vi "VSG25_AM.vi"(0 "Device Handle In":i32, 1 "Run as Subpanel":bool, 2 "AM Cluster In":T1={"Carrier Freq"=1.0, "Baseband Freq"=1.0, "Carrier Hz"=3, "Baseband Hz"=1, "Modulation Depth"=50.0, "Amplitude"=-10.0, "Modulation Shape"=0} {"Modulation Shape" items=["Sine Wave", "Triangle Wave", "Square Wave", "Ramp Wave"]; "Carrier Hz" items=["Hz", "kHz", "MHz", "GHz"]; "Baseband Hz" items=["Hz", "kHz", "MHz", "GHz"]}, 3 "Error In":errorcluster) -> (5 "Device Handle Out":i32, 6 "AM Cluster Out":T1 {"Modulation Shape" items=["Sine Wave", "Triangle Wave", "Square Wave", "Ramp Wave"]; "Carrier Hz" items=["Hz", "kHz", "MHz", "GHz"]; "Baseband Hz" items=["Hz", "kHz", "MHz", "GHz"]}, 7 "Error Out":errorcluster)   [LabVIEW 2014]
uses:
  Frequency Hertz.ctl
  Shape Control.ctl
  AM Cluster.ctl
  sg_lib/VSG25A.lvlib
panel:
  in  "Stop":bool
  out "Device Selected":bool
  in  "Modulation Shape":T3 items=["Sine Wave", "Triangle Wave", "Square Wave", "Ramp Wave"]
  in  "Modulation Depth":dbl
  in  "Baseband Hz":T2 items=["Hz", "kHz", "MHz", "GHz"]
  in  "Baseband Frequency":dbl
  in  "RF On":bool
  in  "Carrier Hz":T2 items=["Hz", "kHz", "MHz", "GHz"]
  in  "Amplitude (dBm)":dbl
  in  "Carrier Frequency":dbl
  # "Amplitude Modulation"
  # "( 1 to 99 %)"
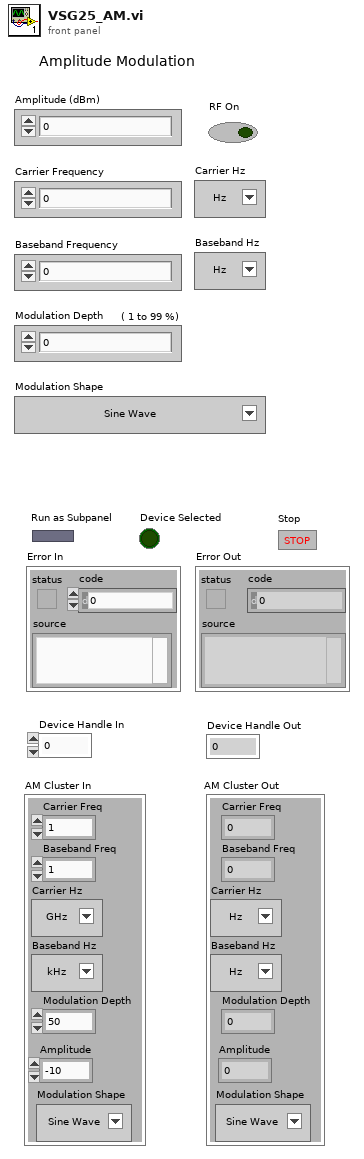
[diagram p1: front panel]
types:
  T1 = typedef "AM Cluster.ctl" = cluster{"Carrier Freq":dbl, "Baseband Freq":dbl, "Carrier Hz":T2, "Baseband Hz":T2, "Modulation Depth":dbl, "Amplitude":dbl, "Modulation Shape":T3}
  T2 = typedef "Frequency Hertz.ctl" = u16
  T3 = typedef "Shape Control.ctl" = u16
  T4 = enum16{"Init", "Proc Events", "Write VSG25", "Exit"}
  T5 = enum32{"Bad", "Idle", "Run top level", "Running"}
  T6 = enum16{"Check Amplitude ", "Check Carrier", "Check Baseband", "Check Modulation Depth", "Stop RF", "Set Freq and Amp", "Set AM", "Finish"}
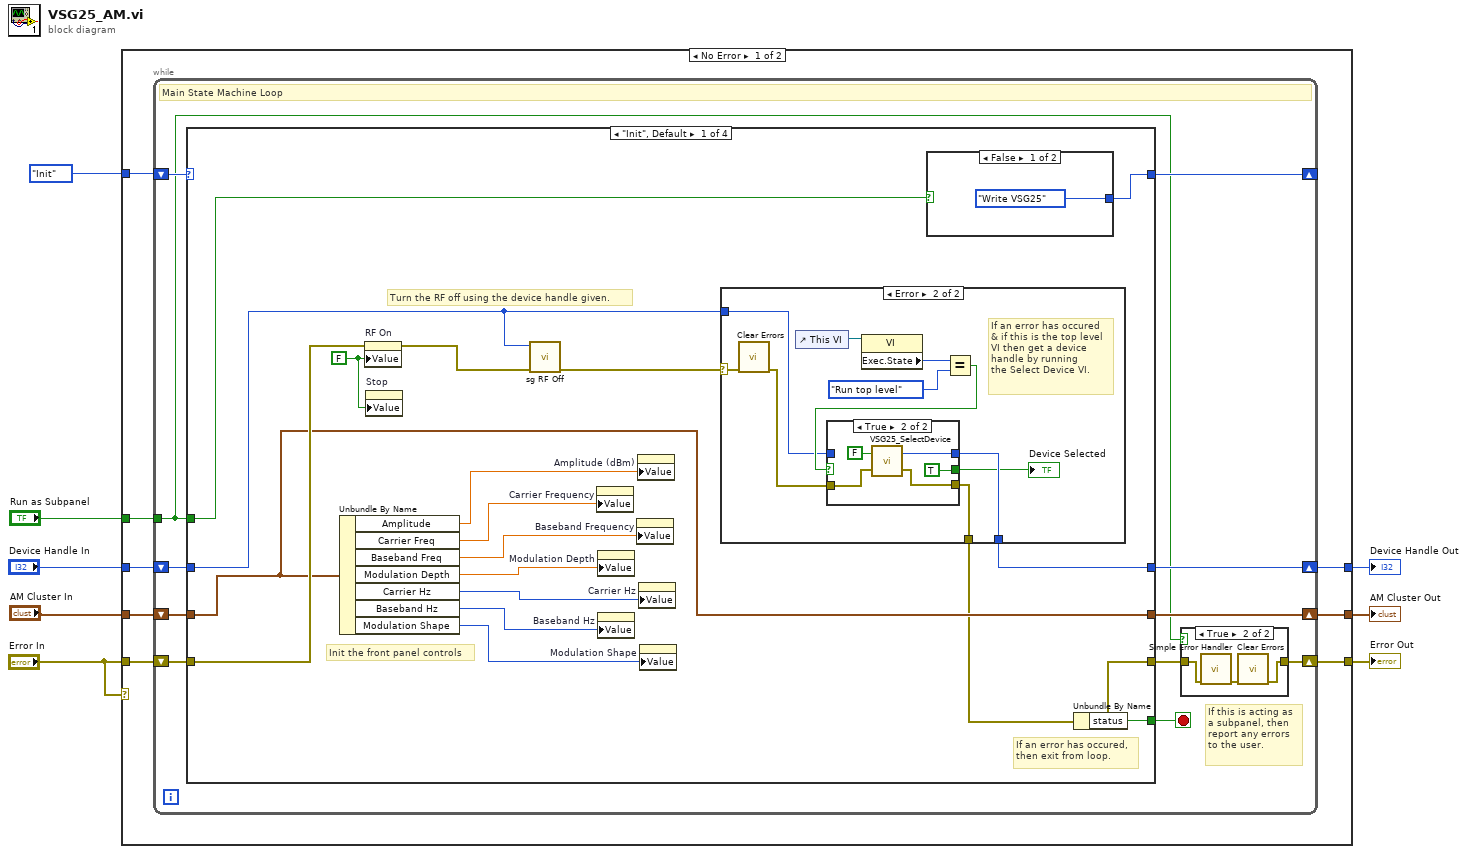
[diagram p0: block diagram]
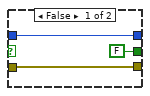
[diagram p4: hidden frame]
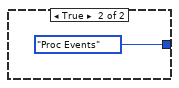
[diagram p5: hidden frame]
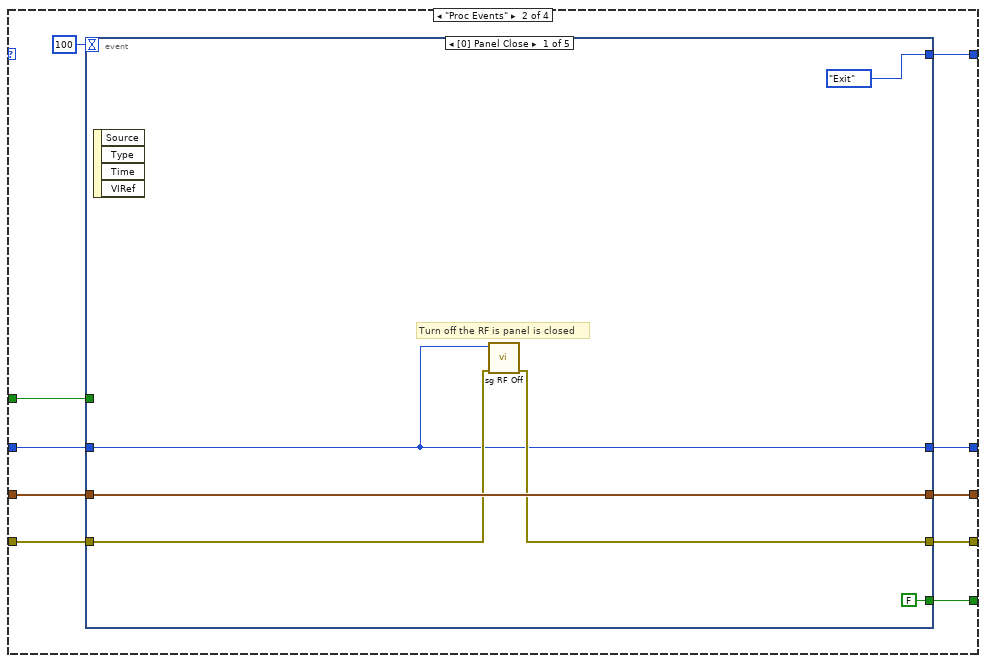
[diagram p6: hidden frame]
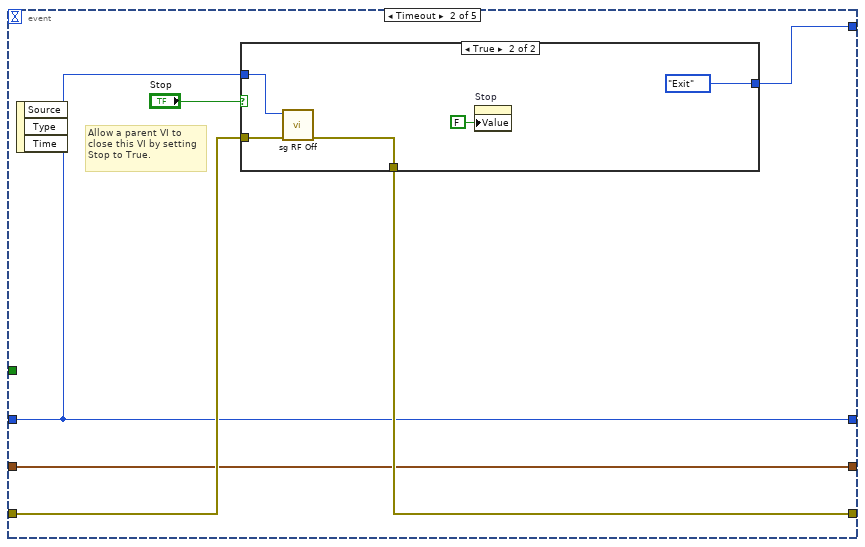
[diagram p7: hidden frame]
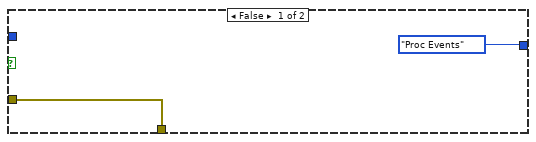
[diagram p8: hidden frame]
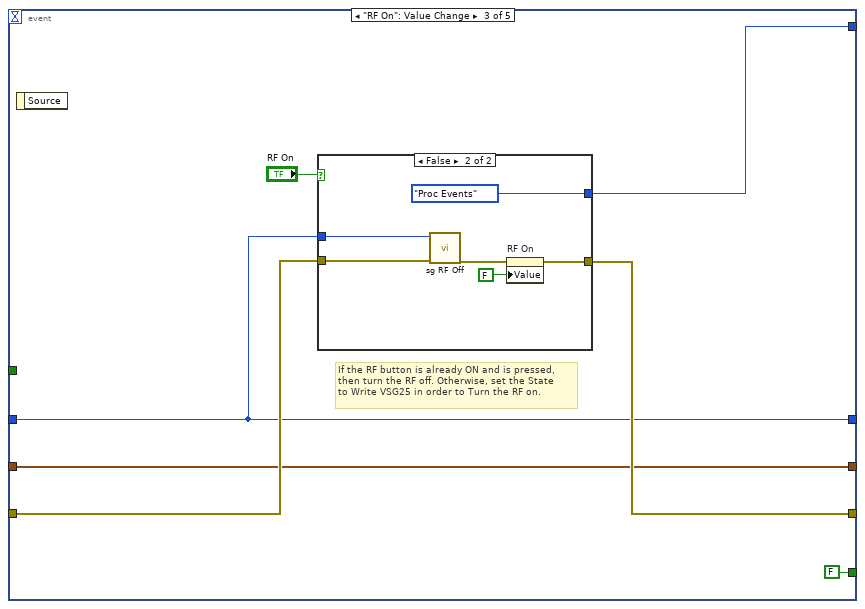
[diagram p9: hidden frame]
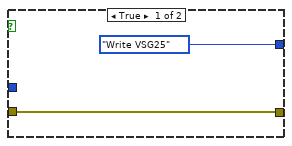
[diagram p10: hidden frame]
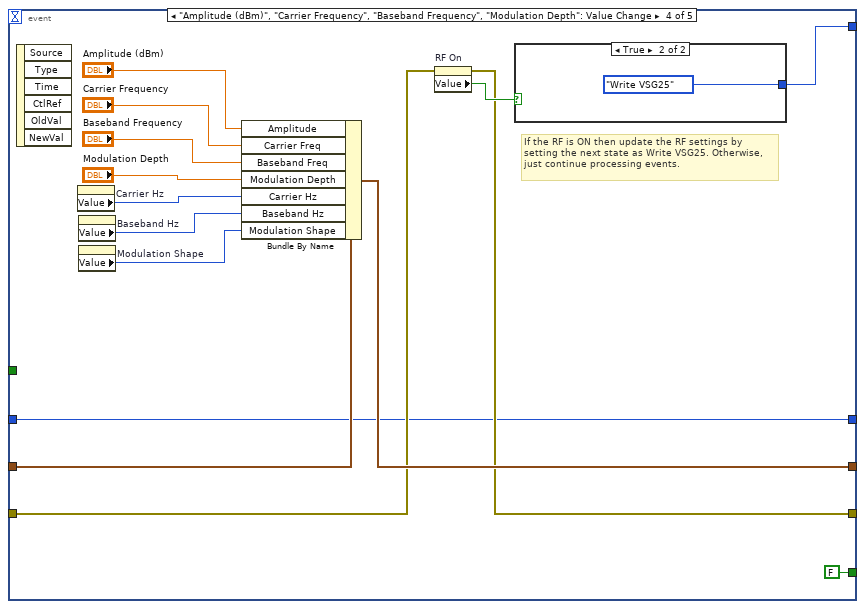
[diagram p11: hidden frame]
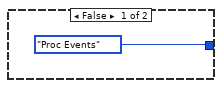
[diagram p12: hidden frame]
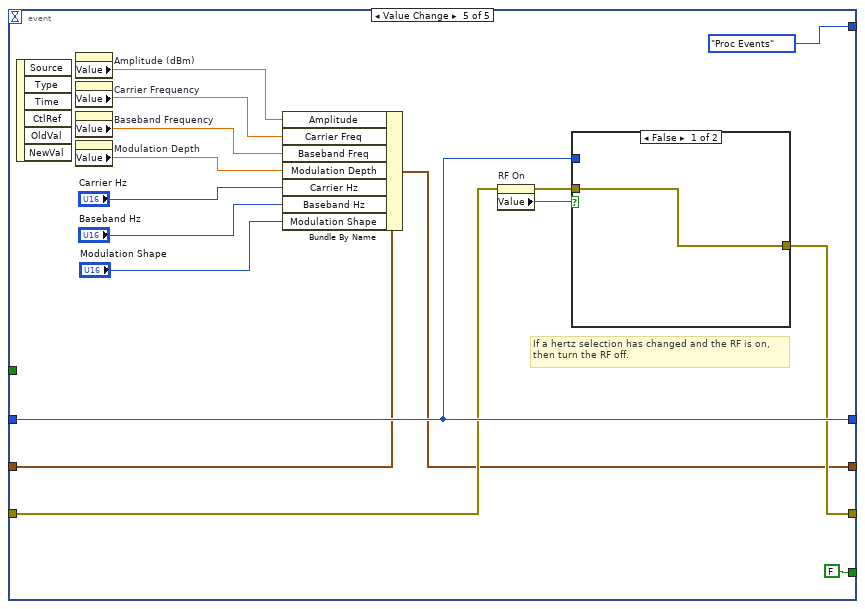
[diagram p13: hidden frame]
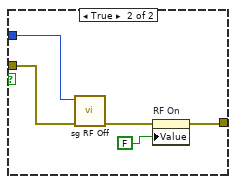
[diagram p14: hidden frame]
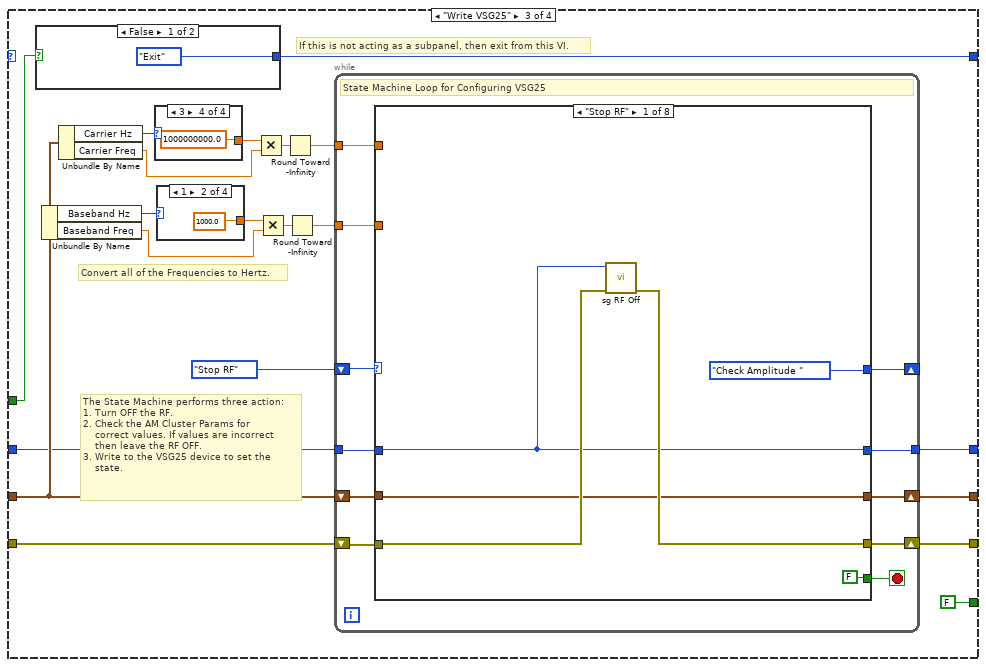
[diagram p15: hidden frame]
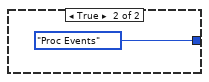
[diagram p16: hidden frame]
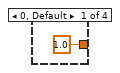
[diagram p17: hidden frame]
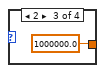
[diagram p18: hidden frame]
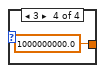
[diagram p19: hidden frame]
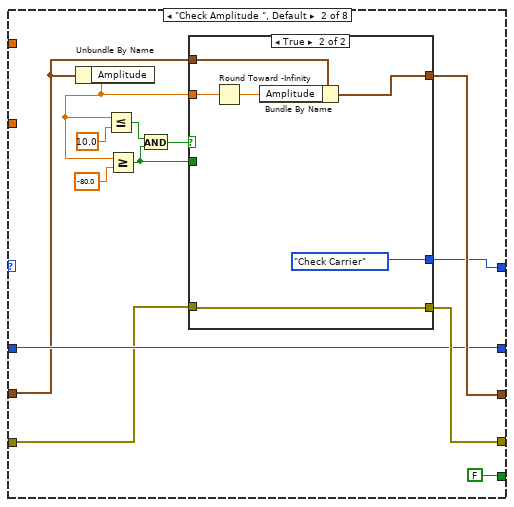
[diagram p20: hidden frame]
diagram:
  n1 = case shown="No Error" "Error In" {
    tunnel: "Error In" -> [w12 w323]
    tunnel: T4."Init" -> [w16 _]
    tunnel: "Run as Subpanel" -> [w15 _]
    tunnel: "Device Handle In" -> [w14 w321]
    tunnel: "AM Cluster In" -> [w13 w322]
    tunnel: [w11 w323] -> w4
    tunnel: [w10 w322] -> w1
    tunnel: [w9 w321] -> w3
    frame No Error {
      n2 = while {
        shift-right: [w26] -> _
        shift-left: w16 -> [w27]
        tunnel: w15 -> [w17]
        shift-right: [w18] -> w11
        shift-left: w12 -> [w23]
        shift-right: [w21] -> w10
        shift-left: w13 -> [w24]
        shift-right: [w20] -> w9
        shift-left: w14 -> [w25]
        stop <- w22 stop-if-true
        # "If this is acting as \na subpanel, then\nreport any errors\nto the user."
        # "Main State Machine Loop"
        n3 = case shown="\"Init\", Default" w27 {
          selector: w27 -> [_ _ _ w316]
          tunnel: [w42 w74 w157 w316] -> w26
          tunnel: w17 -> [w45 w78 w156 _]
          tunnel: w25 -> [w36 w79 w162 w311]
          tunnel: w24 -> [w43 w80 w163 w312]
          tunnel: w23 -> [w44 w81 w166 w313]
          tunnel: [w41 w75 FALSE TRUE] -> w22
          tunnel: [w37 w73 w161 w314] -> w19
          tunnel: [w43 w77 w160 w312] -> w21
          tunnel: [w38 w76 w159 w311] -> w20
          frame "Init", Default {
            w32 = FALSE ("RF On")
            # "Init the front panel controls"
            # "Turn the RF off using the device handle given."
            # "If an error has occured,\nthen exit from loop."
            n4 = Unbundle By Name(w43) -> ("Amplitude"=w49:dbl, "Carrier Freq"=w48:dbl, "Baseband Freq"=w47:dbl, "Modulation Depth"=w46:dbl, "Carrier Hz"=w35:T2, "Baseband Hz"=w34:T2, "Modulation Shape"=w33:T3)
            n5 = property on="RF On" class="Bool (strict)"(error in=w44, "Value"=w32) -> (error out=w40:errorcluster)  [unwired: 1 in, 1 out]
            n6 = property on="Stop" class="Bool (strict)"("Value"=w32) -> ()  [unwired: 2 in, 2 out]
            n7 = call "sg RF Off.vi"("error in (no error)"=w40, "device"=w36) -> ("error out"=w39:errorcluster)  [unwired: 8 in, 1 out]
            n8 = property on="Carrier Frequency" class="DigNum (strict)"("Value"=w48) -> ()  [unwired: 2 in, 2 out]
            n9 = property on="Modulation Depth" class="DigNum (strict)"("Value"=w46) -> ()  [unwired: 2 in, 2 out]
            n10 = property on="Baseband Hz" class="Ring (strict)"("Value"=w34) -> ()  [unwired: 2 in, 2 out]
            n11 = property on="Baseband Frequency" class="DigNum (strict)"("Value"=w47) -> ()  [unwired: 2 in, 2 out]
            n12 = property on="Amplitude (dBm)" class="DigNum (strict)"("Value"=w49) -> ()  [unwired: 2 in, 2 out]
            n13 = property on="Carrier Hz" class="Ring (strict)"("Value"=w35) -> ()  [unwired: 2 in, 2 out]
            n14 = property on="Modulation Shape" class="Ring (strict)"("Value"=w33) -> ()  [unwired: 2 in, 2 out]
            n15 = case shown="Error" w39 {
              selector: w39 -> [w50 w57]
              tunnel: [w51 w55] -> w38
              tunnel: [w50 w54] -> w37
              tunnel: w36 -> [w51 w53]
              frame No Error {
              }
              frame Error {
                # "If an error has occured\n& if this is the top level\nVI then get a device\nhandle by running \nthe Select Device VI."
                n16 = call <vilib>:"Clear Errors.vi"("error in (no error)"=w57) -> ("error out"=w56:errorcluster)  [unwired: 5 in, 1 out]
                n17 = control-ref of="This VI"() -> (w61:refnum<vi>)
                n18 = property class="VI"(reference=w61) -> ("Exec.State"=w60:T5)  [unwired: 1 in, 2 out]
                n19 = Equal?(x=w60, y=T5."Run top level" ("Execution:State 2")) -> (x = y?=w58:bool)
                n20 = case shown="True" w58 {
                  tunnel: [w64 w69] -> w55
                  tunnel: w53 -> [w64 _]
                  tunnel: w56 -> [w63 w67]
                  tunnel: [w63 w66] -> w54
                  tunnel: [FALSE TRUE] -> w52
                  frame False {
                  }
                  frame True {
                    n21 = call "VSG25_SelectDevice.vi"("ErrorIn"=w67, "AutoSel"=FALSE) -> ("ErrorOut"=w66:errorcluster, "deviceHandle"=w69:i32)
                  }
                }
                "Device Selected" <- w52
              }
            }
            n22 = case shown="False" w45 {
              tunnel: [T4."Write VSG25" T4."Proc Events"] -> w42
              frame False {
              }
              frame True {
              }
            }
            n23 = Unbundle By Name(w37) -> ("status"=w41:bool)
          }
          frame "Proc Events" {
            n24 = event shown="[0] Panel Close" {
              selector: _ -> [_ _ _ _ _]
              dyn-events: _ -> [_ _ _ _ _]
              timeout: 100 -> [_ _ _ _ _]
              tunnel: w81 -> [w84 w93 w106 w120 w144]
              tunnel: w80 -> [w85 w91 w104 w130 w143]
              tunnel: w79 -> [w82 w90 w103 w118 w146]
              tunnel: w78 -> [_ _ _ _ _]
              tunnel: [w83 w92 w105 w119 w145] -> w73
              tunnel: [w85 w91 w104 w129 w142] -> w77
              tunnel: [w82 w90 w103 w118 w146] -> w76
              tunnel: [FALSE _ FALSE FALSE FALSE] -> w75
              tunnel: [T4."Exit" w88 w102 w121 T4."Proc Events"] -> w74
              event Panel Close {
                # "Turn off the RF is panel is closed"
                n25 = event-data() -> ()  [unwired: 1 in, 4 out]
                n26 = call "sg RF Off.vi"("error in (no error)"=w84, "device"=w82) -> ("error out"=w83:errorcluster)  [unwired: 8 in, 1 out]
              }
              event Timeout {
                # "Allow a parent VI to \nclose this VI by setting\nStop to True."
                n27 = event-data() -> ()  [unwired: 1 in, 3 out]
                n28 = case shown="True" "Stop" {
                  tunnel: w93 -> [w95 w100]
                  tunnel: [w95 w99] -> w92
                  tunnel: w90 -> [_ w98]
                  tunnel: [T4."Proc Events" T4."Exit"] -> w88
                  frame False {
                  }
                  frame True {
                    n29 = call "sg RF Off.vi"("error in (no error)"=w100, "device"=w98) -> ("error out"=w99:errorcluster)  [unwired: 8 in, 1 out]
                    n30 = property on="Stop" class="Bool (strict)"("Value"=FALSE ("Stop")) -> ()  [unwired: 2 in, 2 out]
                  }
                }
              }
              event "RF On": Value Change {
                # "If the RF button is already ON and is pressed, \nthen turn the RF off. Otherwise, set the State\nto Write VSG25 in order to Turn the RF on."
                n31 = event-data() -> ()  [unwired: 1 in, 1 out]
                n32 = case shown="False" "RF On" {
                  tunnel: [w108 w113] -> w105
                  tunnel: w106 -> [w108 w115]
                  tunnel: w103 -> [_ w114]
                  tunnel: [T4."Write VSG25" T4."Proc Events"] -> w102
                  frame True {
                  }
                  frame False {
                    n33 = call "sg RF Off.vi"("error in (no error)"=w115, "device"=w114) -> ("error out"=w112:errorcluster)  [unwired: 8 in, 1 out]
                    n34 = property on="RF On" class="Bool (strict)"(error in=w112, "Value"=FALSE ("RF On")) -> (error out=w113:errorcluster)  [unwired: 1 in, 1 out]
                  }
                }
              }
              event "Amplitude (dBm)", "Carrier Frequency", "Baseband Frequency", "Modulation Depth": Value Change {
                # "If the RF is ON then update the RF settings by\nsetting the next state as Write VSG25. Otherwise,\njust continue processing events."
                n35 = event-data() -> ()  [unwired: 1 in, 6 out]
                n36 = property on="Carrier Hz" class="Ring (strict)"() -> ("Value"=w124:T2)  [unwired: 2 in, 2 out]
                n37 = property on="Baseband Hz" class="Ring (strict)"() -> ("Value"=w123:T2)  [unwired: 2 in, 2 out]
                n38 = property on="Modulation Shape" class="Ring (strict)"() -> ("Value"=w116:T3)  [unwired: 2 in, 2 out]
                n39 = Bundle By Name(cluster=w130, "Amplitude"="Amplitude (dBm)", "Carrier Freq"="Carrier Frequency", "Baseband Freq"="Baseband Frequency", "Modulation Depth"="Modulation Depth", "Carrier Hz"=w124, "Baseband Hz"=w123, "Modulation Shape"=w116) -> (w129:T1)
                n40 = property on="RF On" class="Bool (strict)"(error in=w120) -> (error out=w119:errorcluster, "Value"=w122:bool)  [unwired: 1 in, 1 out]
                n41 = case shown="True" w122 {
                  tunnel: [T4."Proc Events" T4."Write VSG25"] -> w121
                  frame False {
                  }
                  frame True {
                  }
                }
              }
              event Value Change {
                # "If a hertz selection has changed and the RF is on,\nthen turn the RF off."
                n42 = event-data() -> ()  [unwired: 1 in, 6 out]
                n43 = property on="Amplitude (dBm)" class="DigNum (strict)"() -> ("Value"=w141:dbl)  [unwired: 2 in, 2 out]
                n44 = property on="Carrier Frequency" class="DigNum (strict)"() -> ("Value"=w140:dbl)  [unwired: 2 in, 2 out]
                n45 = property on="Baseband Frequency" class="DigNum (strict)"() -> ("Value"=w139:dbl)  [unwired: 2 in, 2 out]
                n46 = property on="Modulation Depth" class="DigNum (strict)"() -> ("Value"=w138:dbl)  [unwired: 2 in, 2 out]
                n47 = Bundle By Name(cluster=w143, "Amplitude"=w141, "Carrier Freq"=w140, "Baseband Freq"=w139, "Modulation Depth"=w138, "Carrier Hz"="Carrier Hz", "Baseband Hz"="Baseband Hz", "Modulation Shape"="Modulation Shape") -> (w142:T1)
                n48 = property on="RF On" class="Bool (strict)"(error in=w144) -> (error out=w148:errorcluster, "Value"=w147:bool)  [unwired: 1 in, 1 out]
                n49 = case shown="False" w147 {
                  tunnel: [w149 w150] -> w145
                  tunnel: w148 -> [w149 w154]
                  tunnel: w146 -> [_ w153]
                  frame False {
                  }
                  frame True {
                    n50 = call "sg RF Off.vi"("error in (no error)"=w154, "device"=w153) -> ("error out"=w151:errorcluster)  [unwired: 8 in, 1 out]
                    n51 = property on="RF On" class="Bool (strict)"(error in=w151, "Value"=FALSE ("RF On")) -> (error out=w150:errorcluster)  [unwired: 1 in, 1 out]
                  }
                }
              }
            }
          }
          frame "Write VSG25" {
            # "If this is not acting as a subpanel, then exit from this VI."
            # "Convert all of the Frequencies to Hertz."
            # "The State Machine performs three action:\n1. Turn OFF the RF.\n2. Check the AM Cluster Params for \n    correct values. If values are incorrect\n    then leave the RF OFF.\n3. Write to the VSG25 device to set the\n    state."
            n52 = case shown="False" w156 {
              tunnel: [T4."Exit" T4."Proc Events"] -> w157
              frame False {
              }
              frame True {
              }
            }
            n53 = Unbundle By Name(w163) -> ("Baseband Hz"=w168:T2, "Baseband Freq"=w170:dbl)
            n54 = Unbundle By Name(w163) -> ("Carrier Hz"=w173:T2, "Carrier Freq"=w171:dbl)
            n55 = case shown="3" w173 {
              tunnel: [1.0 ("y") 1000.0 ("y") 1000000.0 ("y") 1000000000.0 ("y")] -> w172
              frame 0, Default {
              }
              frame 1 {
              }
              frame 2 {
              }
              frame 3 {
              }
            }
            n56 = case shown="1" w168 {
              tunnel: [1.0 ("y") 1000.0 ("y") 1000000.0 ("y") 1000000000.0 ("y")] -> w169
              frame 0, Default {
              }
              frame 1 {
              }
              frame 2 {
              }
              frame 3 {
              }
            }
            n57 = Multiply(x=w172, y=w171) -> (x*y=w174:dbl)
            n58 = Multiply(x=w169, y=w170) -> (x*y=w167:dbl)
            n59 = Round Toward -Infinity(1:w174) -> (0:w165:dbl)
            n60 = Round Toward -Infinity(1:w167) -> (0:w164:dbl)
            n61 = while {
              shift-right: [w183] -> _
              shift-left: T6."Stop RF" -> [w191]
              tunnel: w165 -> [w184]
              tunnel: w164 -> [w181]
              tunnel: w162 -> [w185]
              tunnel: [w182] -> w159
              shift-right: [w187] -> w161
              shift-left: w166 -> [w189]
              shift-right: [w186] -> w160
              shift-left: w163 -> [w190]
              stop <- w188 stop-if-true
              # "State Machine Loop for Configuring VSG25"
              n62 = case shown="\"Stop RF\"" w191 {
                selector: w191 -> [_ _ _ _ _ _ _ w299]
                tunnel: w190 -> [w194 w200 w228 w248 w265 w284 w291 w301]
                tunnel: w189 -> [w196 w199 w231 w250 w269 w286 w297 w302]
                tunnel: [FALSE FALSE FALSE FALSE FALSE FALSE FALSE TRUE] -> w188
                tunnel: [w195 w203 w230 w247 w267 w283 w296 w302] -> w187
                tunnel: [w194 w202 w228 w248 w265 w284 w291 w301] -> w186
                tunnel: w185 -> [w193 w201 w227 w249 w268 w285 w293 w300]
                tunnel: [w193 w201 w227 w249 w268 w285 w293 w300] -> w182
                tunnel: w184 -> [_ _ w233 _ _ w287 _ _]
                tunnel: [T6."Check Amplitude " w198 w232 w246 w266 T6."Set AM" T6."Finish" w299] -> w183
                tunnel: w181 -> [_ _ _ w251 _ _ w294 _]
                frame "Stop RF" {
                  n63 = call "sg RF Off.vi"("error in (no error)"=w196, "device"=w193) -> ("error out"=w195:errorcluster)  [unwired: 8 in, 1 out]
                }
                frame "Check Amplitude ", Default {
                  n64 = Unbundle By Name(w200) -> ("Amplitude"=w205:dbl)
                  n65 = Less Or Equal?(x=w205, y=10.0) -> (x <= y?=w209:bool)
                  n66 = Greater Or Equal?(x=w205, y=-80.0) -> (x >= y?=w206:bool)
                  n67 = And(x=w209, y=w206) -> (x .and. y?=w210:bool)
                  n68 = case shown="True" w210 {
                    tunnel: w206 -> [w220 _]
                    tunnel: w205 -> [_ w225]
                    tunnel: w200 -> [w217 w224]
                    tunnel: [w216 w223] -> w202
                    tunnel: [T6."Finish" T6."Check Carrier"] -> w198
                    tunnel: w199 -> [w214 w222]
                    tunnel: [w212 w222] -> w203
                    frame False {
                      n69 = Select(t=10.0, s=w220, f=-80.0) -> (s? t:f=w215:dbl)
                      n70 = Bundle By Name(cluster=w217, "Carrier Freq"=w215) -> (w216:T1)
                      n71 = property on="Amplitude (dBm)" class="DigNum (strict)"("Value"=w215) -> ()  [unwired: 2 in, 2 out]
                      n72 = Merge Errors(w214, errorcluster {"status"=TRUE, "code"=-1, "source"="Invalid Amplitude.\nValue must be between\n-80 dBm and 10 dBm."} ("error constant")) -> (w212:errorcluster)
                    }
                    frame True {
                      n73 = Round Toward -Infinity(1:w225) -> (0:w226:dbl)
                      n74 = Bundle By Name(cluster=w224, "Amplitude"=w226) -> (w223:T1)
                    }
                  }
                }
                frame "Check Carrier" {
                  n75 = Greater Or Equal?(x=w233, y=80000000.0) -> (x >= y?=w234:bool)
                  n76 = Less Or Equal?(x=w233, y=2500000000.0) -> (x <= y?=w238:bool)
                  n77 = Compound Arithmetic op=AND(w234, w238) -> (w235:bool)
                  n78 = case shown="True" w235 {
                    tunnel: [T6."Finish" T6."Check Baseband"] -> w232
                    tunnel: w231 -> [w241 w244]
                    tunnel: [w242 w244] -> w230
                    frame False {
                      n79 = Merge Errors(w241, errorcluster {"status"=TRUE, "code"=-1, "source"="Carrier frequency must \nbe greater than 80 MHz\nand less than 2.5 GHz."} ("error constant")) -> (w242:errorcluster)
                    }
                    frame True {
                    }
                  }
                }
                frame "Check Baseband" {
                  n80 = Greater Or Equal?(x=w251, y=30.0) -> (x >= y?=w252:bool)
                  n81 = Less Or Equal?(x=w251, y=40000000.0) -> (x <= y?=w256:bool)
                  n82 = Compound Arithmetic op=AND(w252, w256) -> (w253:bool)
                  n83 = case shown="True" w253 {
                    tunnel: [T6."Finish" T6."Check Modulation Depth"] -> w246
                    tunnel: w250 -> [w260 w262]
                    tunnel: [w258 w262] -> w247
                    frame False {
                      n84 = Merge Errors(w260, errorcluster {"status"=TRUE, "code"=-1, "source"="Baseband frequency must \nbe greater than 30 Hz\nand less than 40 MHz."} ("error constant")) -> (w258:errorcluster)
                    }
                    frame True {
                    }
                  }
                }
                frame "Check Modulation Depth" {
                  n85 = Unbundle By Name(w265) -> ("Modulation Depth"=w264:dbl)
                  n86 = Greater Or Equal?(x=w264, y=1.0) -> (x >= y?=w270:bool)
                  n87 = Less Or Equal?(x=w264, y=99.0) -> (x <= y?=w274:bool)
                  n88 = Compound Arithmetic op=AND(w270, w274) -> (w271:bool)
                  n89 = case shown="True" w271 {
                    tunnel: [T6."Finish" T6."Set Freq and Amp"] -> w266
                    tunnel: w269 -> [w277 w280]
                    tunnel: [w278 w280] -> w267
                    frame False {
                      n90 = Merge Errors(w277, errorcluster {"status"=TRUE, "code"=-1, "source"="Modulation Depth must \nbe greater than 1 and less \nthan 99 percent."} ("error constant")) -> (w278:errorcluster)
                    }
                    frame True {
                    }
                  }
                }
                frame "Set Freq and Amp" {
                  n91 = Unbundle By Name(w284) -> ("Amplitude"=w288:dbl)
                  n92 = call "sg Set Frequency Amplitude.vi"("error in (no error)"=w286, "amplitude"=w288, "frequency"=w287, "device"=w285) -> ("error out"=w283:errorcluster)  [unwired: 6 in, 1 out]
                }
                frame "Set AM" {
                  n93 = Unbundle By Name(w291) -> ("Modulation Shape"=w292:T3, "Modulation Depth"=w290:dbl)
                  n94 = call "sg Set AM.vi"("shape"=w292, "error in (no error)"=w297, "depth"=w290, "frequency"=w294, "device"=w293) -> ("error out"=w296:errorcluster)  [unwired: 5 in, 1 out]
                }
                frame "Finish" {
                  # "If no errors have occured, then indicate that the RF is ON."
                  n95 = case shown="No Error" w302 {
                    tunnel: [TRUE FALSE] -> w303
                    frame No Error {
                    }
                    frame Error {
                    }
                  }
                  n96 = property on="RF On" class="Bool (strict)"("Value"=w303) -> ()  [unwired: 2 in, 2 out]
                }
              }
            }
          }
          frame "Exit" {
            # "If a device handle was\nacquired using the \nSelect Device VI, then\nclose the handle \nbefore exiting."
            n97 = local read "Device Selected"() -> (w310:bool)
            n98 = case shown="True" w310 {
              tunnel: w311 -> [_ w320]
              tunnel: w313 -> [w317 w319]
              tunnel: [w317 w318] -> w314
              frame False {
              }
              frame True {
                n99 = call "sg Close Device.vi"("error in (no error)"=w319, "device"=w320) -> ("error out"=w318:errorcluster)  [unwired: 8 in, 1 out]
              }
            }
          }
        }
        n100 = case shown="True" w17 {
          tunnel: w19 -> [w28 w30]
          tunnel: [w28 w31] -> w18
          frame False {
          }
          frame True {
            n101 = call <vilib>:"Simple Error Handler.vi"("error in (no error)"=w30) -> ("error out"=w29:errorcluster)  [unwired: 4 in, 4 out]
            n102 = call <vilib>:"Clear Errors.vi"("error in (no error)"=w29) -> ("error out"=w31:errorcluster)  [unwired: 5 in, 1 out]
          }
        }
      }
    }
    frame Error {
    }
  }
  "Error Out" <- w4
  "Device Handle Out" <- w3
  "AM Cluster Out" <- w1
